vi "FTW-dotNET-SQL-OpenConnection.vi"(5 "Connection String":string, 11 "error in":errorcluster) -> (4 "DB Connection":refnum<k24>, 8 "ServerVersion":string, 15 "error out":errorcluster)   [LabVIEW 2015]
uses:
  System.Data
panel:
  # "Inputs"
  # "Outputs"
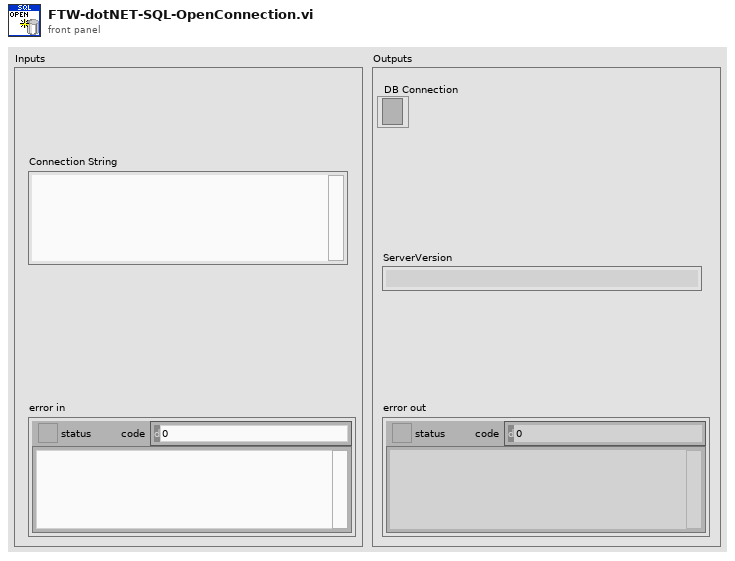
[diagram p1: front panel]
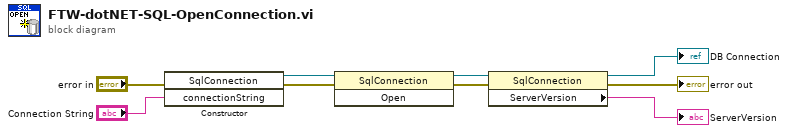
[diagram p0: block diagram]
diagram:
  n1 = constructor class="SqlConnection"(error in="error in", "connectionString"="Connection String") -> (reference out=w9:refnum<k24>, error out=w7:errorcluster)  [unwired: 2 in, 2 out]
  n2 = invoke class="SqlConnection" method="Open"(reference=w9, error in=w7) -> (reference out=w8:refnum<k24>, error out=w6:errorcluster)  [unwired: 1 in, 1 out]
  n3 = property class="SqlConnection"(reference=w8, error in=w6) -> (reference out=→"DB Connection":refnum<k24>, error out=→"error out":errorcluster, "ServerVersion"=→"ServerVersion":string)
